vi "Decode Parallel Schedule Message.vi"(8 "error in (no error)":errorcluster, 10 "Schedule message - parallel":T1={"Schedules"=[], "Synchronised"=[{"Status"=FALSE, "FPGA Name"=""}]}, 11 "Tamer in":refnum<class "Tamer.lvclass">) -> (0 "error out":errorcluster, 3 "Tamer out":refnum<class "Tamer.lvclass">)   [LabVIEW 2020, in "TALOS.lvlib" / "Tamer.lvlib" / "Tamer.lvclass"]
uses:
  Tamer.lvclass
  Run Utilities/TypeDefs/Messages/Schedule Message - Parallel.ctl
  Run Utilities/Schedule/Schedule.lvclass
  Run Utilities/TypeDefs/Synchronize FPGA Cluster.ctl
  Run Utilities/TypeDefs/Monkey Status.ctl
  Tamer.lvclass/Tamer.ctl
  Ancestor/Ancestor/Ancestor.lvclass/Ancestor.ctl
  FGV/Error Memory/Get Error Description.vi
  Support VIs/Get PC name.vi
  Ancestor/Ancestor/Read ID.vi
  Support VIs/Get Class Name.vi
  <vilib>/Utility/error.llb/Clear Errors.vi
  FGV/Error Memory/Error Memory Core.vi
  <vilib>/AdvancedString/Delimited String to 1D String Array.vi
  Support VIs/Circus Root Path.vi
  FGV/Error Memory/Error Crt Lvl checker.vi
  FGV/Error Memory/Error Memory Core.vi/40c8088d-b597-4017-91af-faa98e00292e.vi
  FGV/Error Memory/Error Memory Core.vi/d4a3ab98-063c-4e44-b43d-fbdcfe6c2be2.vi
  Support VIs/Global Memory.vi
  <vilib>/Utility/LVClass/Get LV Class Name.vi
  Support VIs/Is in Packed Library.vi
  Support VIs/TALOS Root path.vi
  Support VIs/Read CSV worksheet.vi
  Support VIs/Global Constants.vi
  <vilib>/Utility/error.llb/General Error Handler.vi
  Ancestor/Ancestor/Ancestor.lvclass
  <vilib>/Comparison/Equal/Equal Functor/Equal Functor.lvclass
  TALOS.lvlib
  Run Utilities/Run Utilities.lvlib
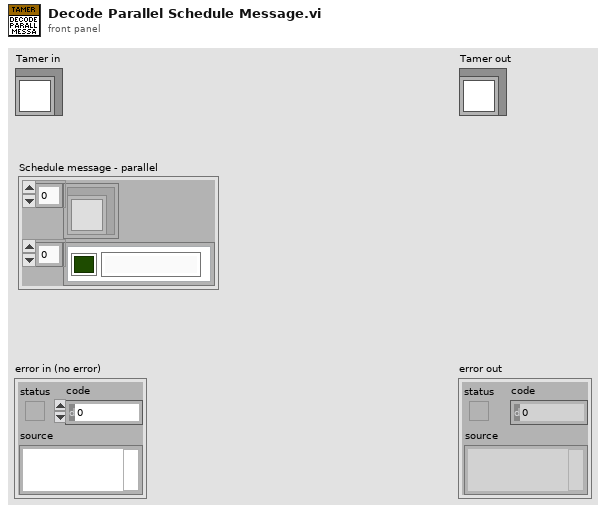
[diagram p1: front panel]
types:
  T1 = typedef "TALOS.lvlib/Run Utilities.lvlib/Schedule Message - Parallel.ctl" = cluster{"Schedules":refnum<class "Schedule.lvclass">[], "Synchronised":T2[]}
  T2 = typedef "TALOS.lvlib/Run Utilities.lvlib/Synchronize FPGA Cluster.ctl" = cluster{"Status":bool, "FPGA Name":string}
  T3 = typedef "TALOS.lvlib/Run Utilities.lvlib/Monkey Status.ctl" = enum16{"Init", "Paused", "Ongoing", "Stopped", "Finished (no errors)", "Finished (with errors)"}
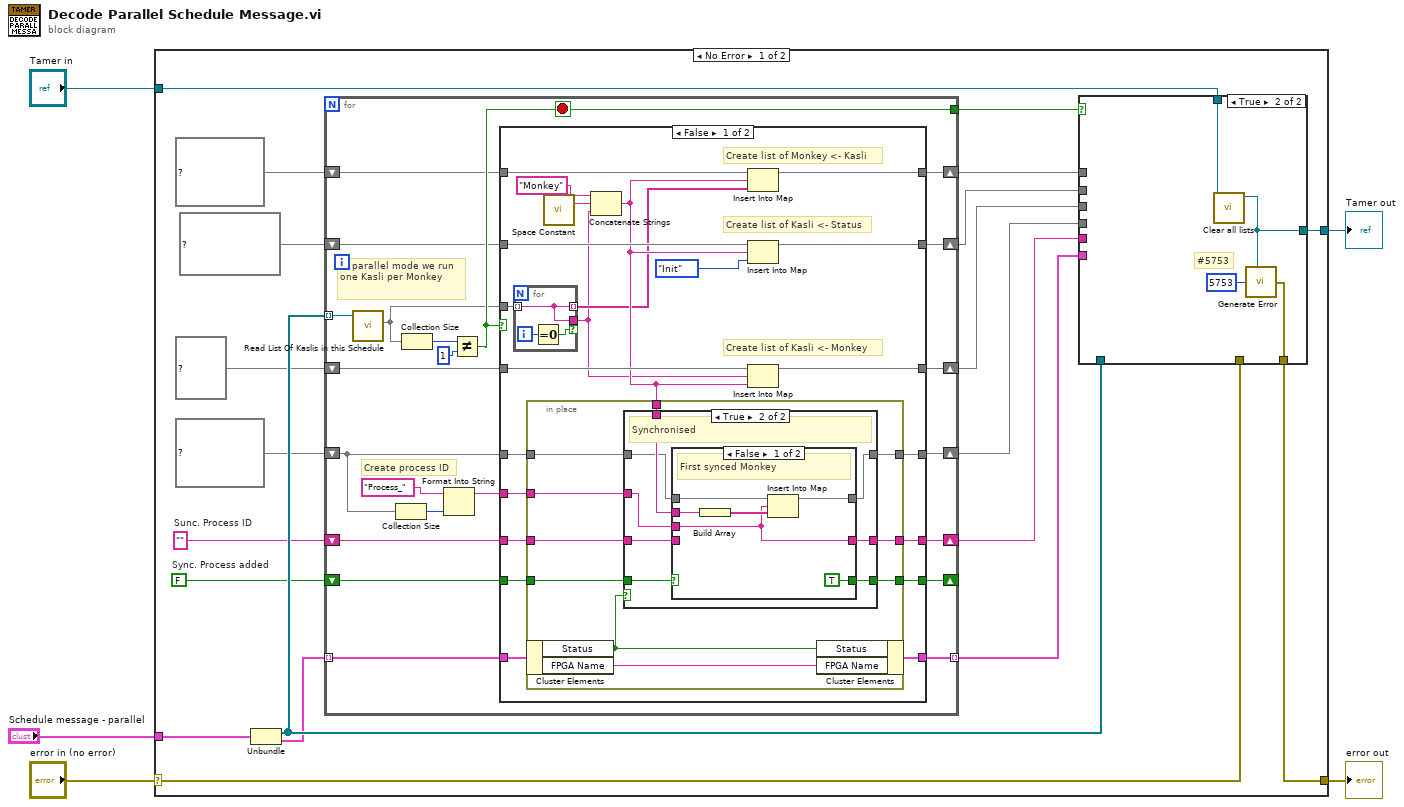
[diagram p0: block diagram]
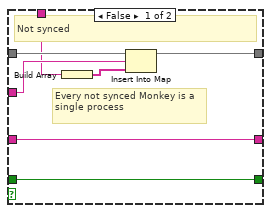
[diagram p2: hidden frame]
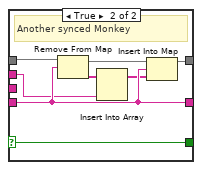
[diagram p3: hidden frame]
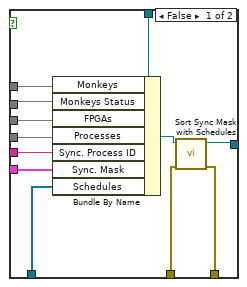
[diagram p5: hidden frame]
diagram:
  n1 = case shown="No Error" "error in (no error)" {
    selector: "error in (no error)" -> [w21 w136]
    tunnel: [w23 w136] -> w4
    tunnel: [w24 w135] -> w2
    tunnel: "Tamer in" -> [w20 w135]
    tunnel: "Schedule message - parallel" -> [w22 _]
    frame No Error {
      w8 = ""  # Sunc. Process ID
      w11 = FALSE  # Sync. Process added
      n2 = Unbundle(w22) -> ("Schedules"=w17:refnum<class "Schedule.lvclass">[], "Synchronised"=w13:T2[])
      n3 = for {
        shift-right: [w45] -> w19
        shift-left: map{string, string[]} {} ("Monkeys") -> [w46]
        tunnel: w17 -> [w44] mode=indexing
        shift-right: [w39] -> w16
        shift-left: map{string, string} {} ("Kaslis") -> [w40]
        tunnel: [w47] -> w18
        shift-right: [w37] -> w14
        shift-left: map{string, T3} {} ("Monkeys Status") -> [w38]
        tunnel: w13 -> [w36] mode=indexing
        tunnel: [w35] -> w6 mode=indexing
        shift-right: [w34] -> w9
        shift-left: map{string, string[]} {} ("Processes") -> [w30]
        shift-right: [w32] -> _
        shift-left: w11 -> [w33]
        shift-right: [w26] -> w7
        shift-left: w8 -> [w28]
        stop <- w47 stop-if-true
        # "Create process ID"
        # "In parallel mode we run one Kasli per Monkey"
        n4 = call-dynamic "Read List Of Kaslis in this Schedule.vi"("Schedule in"=w44) -> ("List of FPGAs"=w41:set{string})  [unwired: 8 in, 2 out]
        n5 = Collection Size(1:w30) -> (0:w31:i32)
        n6 = Collection Size(1:w41) -> (0:w43:i32)
        n7 = Format Into String(initial string="Process_", w31) -> (resulting string=w27:string)  [unwired: 2 in, 1 out]
        n8 = Not Equal?(x=w43, y=1) -> (x != y?=w47:bool)
        n9 = case shown="False" w47 {
          tunnel: w46 -> [w69 w118]
          tunnel: [w68 w118] -> w45
          tunnel: w41 -> [w50 _]
          tunnel: w40 -> [w55 w117]
          tunnel: [w65 w117] -> w39
          tunnel: w38 -> [w64 w116]
          tunnel: [w62 w116] -> w37
          tunnel: w36 -> [w61 w112]
          tunnel: [w60 w112] -> w35
          tunnel: [w59 w115] -> w34
          tunnel: w30 -> [w58 w115]
          tunnel: w33 -> [w57 w114]
          tunnel: [w56 w114] -> w32
          tunnel: w27 -> [w54 _]
          tunnel: w28 -> [w52 w113]
          tunnel: [w51 w113] -> w26
          frame False {
            # "Create list of Kasli <- Monkey"
            # "Create list of Kasli <- Status"
            # "Create list of Monkey <- Kasli"
            n10 = for {
              tunnel: w50 -> [w72] mode=indexing
              tunnel: [w72] -> w49 mode=indexing
              tunnel: [w72] -> w48 if=w70
              i -> [w71]
              n11 = Equal To 0?(x=w71) -> (x = 0?=w70:bool)
            }
            n12 = call <vilib>:"Space Constant.vi"() -> ("String"=w66:string)
            n13 = Concatenate Strings("Monkey" ("string"), w66, w48) -> (w53:string)
            n14 = in-place {
              in-place-border: [w79] -> w59
              in-place-border: w58 -> [w80]
              in-place-border: w57 -> [w76]
              in-place-border: [w75] -> w56
              in-place-border: w54 -> [w81]
              in-place-border: w53 -> [w78]
              in-place-border: w52 -> [w77]
              in-place-border: [w74] -> w51
              n15 = in-place-cluster #1(w61) -> ("Status"=w73:bool, "FPGA Name"=w82:string)
              n16 = case shown="True" w73 {
                tunnel: w81 -> [w87 w93]
                tunnel: w80 -> [w89 w94]
                tunnel: [w88 w92] -> w79
                tunnel: w78 -> [w85 w96]
                tunnel: w77 -> [w84 w90]
                tunnel: w76 -> [w83 w97]
                tunnel: [w83 w95] -> w75
                tunnel: [w84 w91] -> w74
                frame False {
                  # "Every not synced Monkey is a single process"
                  # "Not synced"
                  n17 = Build Array(w85) -> (w86:string[])
                  n18 = Insert Into Map(map in=w89, key=w87, value=w86) -> (map out=w88:map{string, string[]})  [unwired: 2 out]
                }
                frame True {
                  # "Synchronised"
                  n19 = case shown="False" w97 {
                    selector: w97 -> [_ w111]
                    tunnel: [w101 w109] -> w92
                    tunnel: w94 -> [w102 w110]
                    tunnel: w96 -> [w100 w105]
                    tunnel: [TRUE w111] -> w95
                    tunnel: w93 -> [w98 _]
                    tunnel: [w98 w107] -> w91
                    tunnel: w90 -> [_ w107]
                    frame False {
                      # "First synced Monkey"
                      n20 = Build Array(w100) -> (w99:string[])
                      n21 = Insert Into Map(map in=w102, key=w98, value=w99) -> (map out=w101:map{string, string[]})  [unwired: 2 out]
                    }
                    frame True {
                      # "Another synced Monkey"
                      n22 = Remove From Map(10:w107, 11:w110) -> (1:w106:string[], 3:w108:map{string, string[]})  [unwired: 1 out]
                      n23 = Insert Into Array(array=w106, new element=w105) -> (w104:string[])  [unwired: 1 in]
                      n24 = Insert Into Map(map in=w108, key=w107, value=w104) -> (map out=w109:map{string, string[]})  [unwired: 2 out]
                    }
                  }
                }
              }
              n25 = in-place-cluster #1("Status"=w73, "FPGA Name"=w82) -> (w60:T2)
            }
            n26 = Insert Into Map(map in=w69, key=w53, value=w49) -> (map out=w68:map{string, string[]})  [unwired: 2 out]
            n27 = Insert Into Map(map in=w64, key=w53, value=Monkey_Status."Init") -> (map out=w62:map{string, T3})  [unwired: 2 out]
            n28 = Insert Into Map(map in=w55, key=w48, value=w53) -> (map out=w65:map{string, string})  [unwired: 2 out]
          }
          frame True {
          }
        }
      }
      n29 = case shown="True" w18 {
        tunnel: [w122 w131] -> w24
        tunnel: [w119 w134] -> w23
        tunnel: w21 -> [w120 _]
        tunnel: w20 -> [w130 w132]
        tunnel: w19 -> [w129 _]
        tunnel: w17 -> [w126 _]
        tunnel: w16 -> [w128 _]
        tunnel: w14 -> [w127 _]
        tunnel: w6 -> [w125 _]
        tunnel: w9 -> [w124 _]
        tunnel: w7 -> [w123 _]
        frame False {
          n30 = Bundle By Name(cluster=w130, "Monkeys"=w129, "Monkeys Status"=w127, "FPGAs"=w128, "Processes"=w124, "Sync. Process ID"=w123, "Sync. Mask"=w125, "Schedules"=w126) -> (w121:refnum<class "Tamer.lvclass">)
          n31 = call "Sort Sync Mask with Schedules.vi"("error in (no error)"=w120, "Tamer in"=w121) -> ("error out"=w119:errorcluster, "Tamer out"=w122:refnum<class "Tamer.lvclass">)  [unwired: 8 in]
        }
        frame True {
          # "#5753"
          n32 = call-dynamic "Clear all lists.vi"("Tamer in"=w132) -> ("Tamer out"=w131:refnum<class "Tamer.lvclass">)  [unwired: 9 in, 1 out]
          n33 = call "Generate Error.vi"("Class"=w131, "Error Code"=5753) -> ("error out"=w134:errorcluster)  [unwired: 5 in]
        }
      }
    }
    frame Error {
    }
  }
  "error out" <- w4
  "Tamer out" <- w2
